vi "Teardown.vi"(8 "Error in":errorcluster, 9 "Unhandled Msgs":refnum<class "Msg.lvclass">[](array[class]), 10 "Teardown Location":T1, 11 "Actor in":refnum<class "Actor.lvclass">) -> (3 "Actor out":refnum<class "Actor.lvclass">)   [LabVIEW 2025, in "jettl.lvlib" / "Actor.lvlib" / "Actor.lvclass"]
uses:
  Actor.lvclass
  Teardown Location.ctl
  Msg/Msg.lvclass
  Actor.lvlib
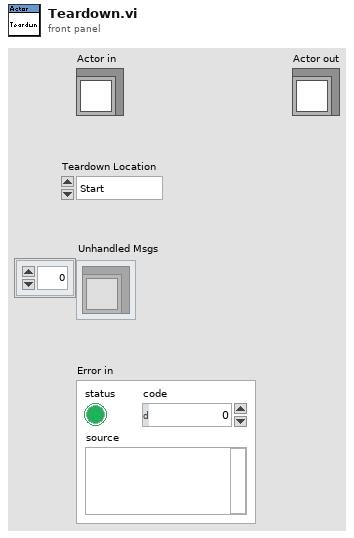
[diagram p1: front panel]
types:
  T1 = typedef "jettl.lvlib/Actor.lvlib/Teardown Location.ctl" = enum16{"Start", "Stop"}
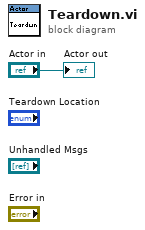
[diagram p0: block diagram]
diagram:
  "Actor out" <- "Actor in"
